vi "624WPI_DashboardGetInfo.vi"(7 "Vision":u16(ring) items=["Camera Off", "USB Camera SW", "USB Camera HW", "IP Camera"], 8 "Binding Refnum":refnum<notifier>, 9 "Window Mode Notifier":refnum<notifier>, 11 "TCP Cnx":refnum<k5>) -> (0 "Power and Errors":T2, 1 "Robot Metrics":T3, 2 "Status Info":T5, 3 "Control Info":T4 {"Team Station" items=["Red 1", "Red 2", "Red 3", "Blue 1", "Blue 2", "Blue 3"]}, 4 "Robot Mode":T1(ring), 5 "Process?":bool, 6 "Custom Dashboard Data":string)   [LabVIEW 2015]
uses:
  Dashboard Hijack Data.ctl
  <vilib>/Rock Robotics/WPI/Dashboard/WPI_DashboardLogging Global.vi
panel:
  # "CAN Metrics\nJS HID Outputs\nFree Mem"
  # "Need to merge in TCP info too"
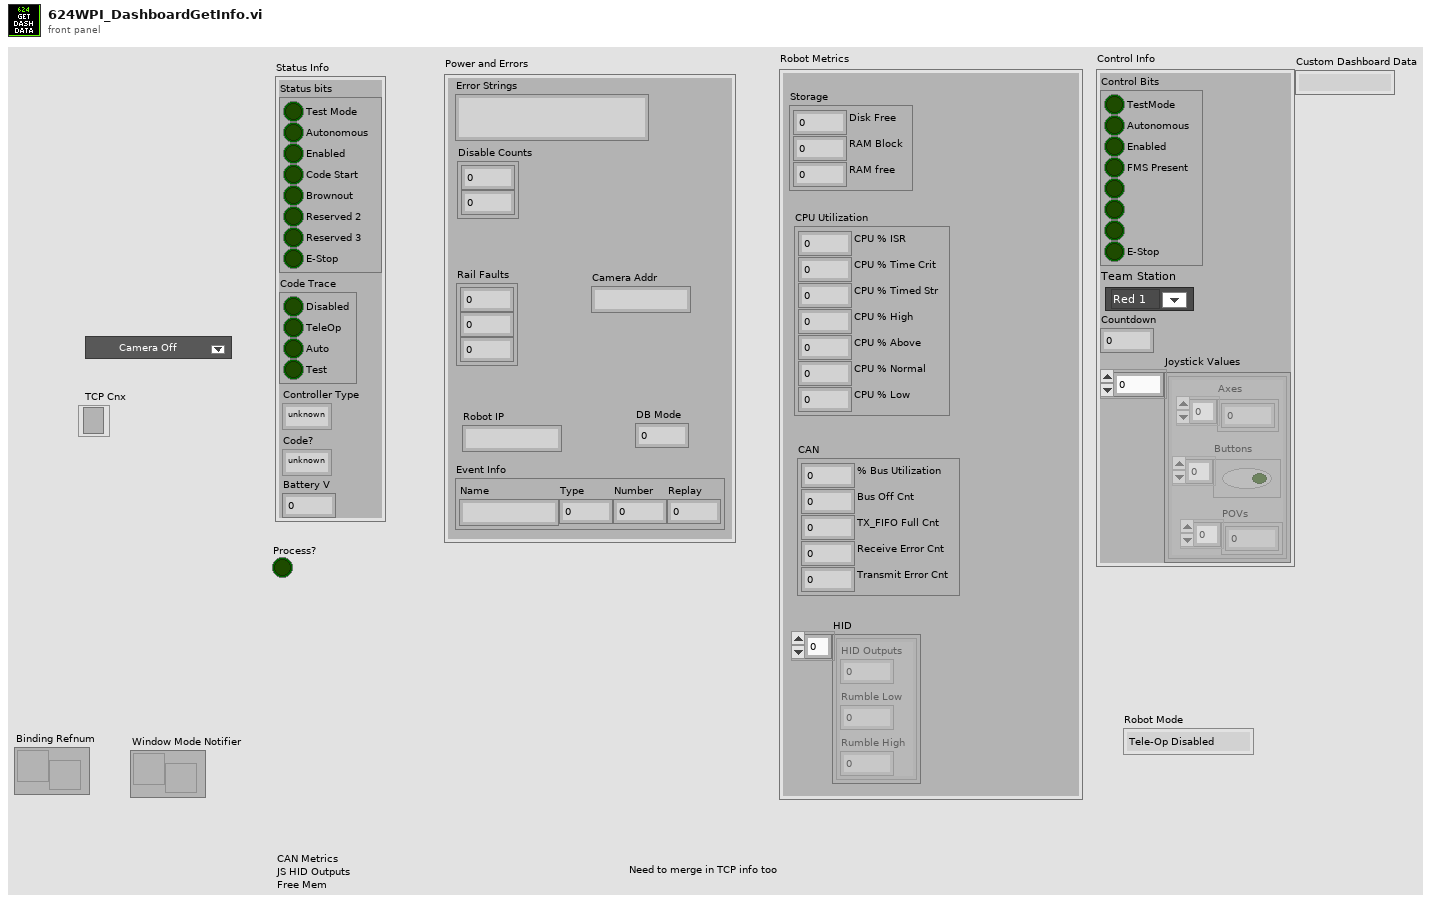
[diagram p1: front panel]
types:
  T1 = enum8{"Tele-Op Disabled", "Tele-Op Enabled", "Auto Disabled", "Auto Enabled", "Test Disabled", "Test Enabled", "Disconnected", "No Code", "E-Stop"}
  T2 = cluster{"Error Strings":string, "Disable Counts":cluster{u16, u16}, "Rail Faults":cluster{u16, u16, u16}, "Robot IP":string, "DB Mode":u8, "Event Info":cluster{"Name":string, "Type":u8, "Number":u16, "Replay":u8}, "Camera Addr":string}
  T3 = cluster{"Storage":cluster{"Disk Free":u64, "RAM Block":u32, "RAM free":u32}, "CPU Utilization":cluster{"CPU % ISR":sgl, "CPU % Time Crit":sgl, "CPU % Timed Str":sgl, "CPU % High":sgl, "CPU % Above":sgl, "CPU % Normal":sgl, "CPU % Low":sgl}, "CAN":cluster{"% Bus Utilization":sgl, "Bus Off Cnt":u32, "TX_FIFO Full Cnt":u32, "Receive Error Cnt":u8, "Transmit Error Cnt":u8}, "HID":cluster{"HID Outputs":u32, "Rumble Low":u16, "Rumble High":u16}[]}
  T4 = cluster{"Control Bits":cluster{"TestMode":bool, "Autonomous":bool, "Enabled":bool, "FMS Present":bool, bool, bool, bool, "E-Stop":bool}, "Team Station ":u8, "Countdown":sgl, "Joystick Values":cluster{"Axes":dbl[], "Buttons":bool[], "POVs":i16[]}[]}
  T5 = cluster{"Status bits":cluster{"Test Mode":bool, "Autonomous":bool, "Enabled":bool, "Code Start":bool, "Brownout":bool, "Reserved 2":bool, "Reserved 3":bool, "E-Stop":bool}, "Code Trace":cluster{"Disabled":bool, "TeleOp":bool, "Auto":bool, "Test":bool}, "Controller Type":enum16{"unknown", "cRIO", "roboRio"}, "Code?":enum16{"unknown", "noCode", "code"}, "Battery V":dbl}
  T6 = typedef "Dashboard Hijack Data.ctl" = cluster{"UDP Status string":string, "Extra data string":string}
  T7 = cluster{"TestMode":bool, "Autonomous":bool, "Enabled":bool, "FMS Present":bool, bool, bool, bool, "E-Stop":bool}
  T8 = enum16{"Standard", "Buffered", "CRLF", "Immediate"}
  T9 = cluster{"UDP Status":string, "TCP":string, "UDP Control":string}
  T10 = cluster{cluster{"Disk Free":u64, "RAM Block":u32, "RAM free":u32}, cluster{"CPU Load ISR":sgl, "CPU Load Time Critical Pr":sgl, "CPU Load Timed Str Pr":sgl, "CPU Load High Pr":sgl, "CPU Load Above Normal Pr":sgl, "CPU Load Normal Pr":sgl, "CPU Load Low Pr":sgl}, cluster{"% Bus Utilization":sgl, "Bus Off Cnt":u32, "TX_FIFO Full Cnt":u32, "Receive Error Cnt":u8, "Transmit Error Cnt":u8}, cluster{"HID Outputs":u32, "Rumble Low":u16, "Rumble High":u16}[]}
  T11 = cluster{"Status":cluster{"Test Mode":bool, "Autonomous":bool, "Enabled":bool, "Code Start":bool, "Brownout":bool, "Reserved 2":bool, "Reserved 3":bool, "E-Stop":bool}, cluster{bool, bool, bool, bool}, "ctrl":enum16{"unknown", "cRIO", "roboRio"}, "code?":enum16{"unknown", "noCode", "code"}, dbl}
  T12 = cluster{"Boolean array":cluster{"Boolean array[0]":bool, "Boolean array[1]":bool, "Boolean array[2]":bool, "Boolean array[3]":bool, "Boolean array[4]":bool, "Boolean array[5]":bool, "Boolean array[6]":bool, "Boolean array[7]":bool}, u8, "Countdown":sgl, cluster{dbl[], bool[], i16[]}[]}
  T13 = cluster{"Error Strings":string, "Disable Counts":cluster{u16, u16}, "Rail Faults":cluster{u16, u16, u16}, "Robot IP":string, "Mode":u8, "Event Info":cluster{"Name":string, "Type":u8, "Number":u16, "Replay":u8}, "Robot IP":string}
  T14 = cluster{"Boolean array[0]":bool, "Boolean array[1]":bool, "Boolean array[2]":bool, "Boolean array[3]":bool, "Boolean array[4]":bool, "Boolean array[5]":bool, "Boolean array[6]":bool, "Boolean array[7]":bool}
  T15 = typedef "Protocol Operations.ctl" = enum16{"Unknown", "Keep Alive", "Client Hello", "Version not supported", "Server Hello Complete", "Assign", "Update", "No Op", "Server Hello", "Client Hello Complete", "Update Flags", "Delete Entry", "Delete All", "RPC Exec", "RPC Response"}
  T16 = typedef "Field Data.ctl" = cluster{"Dbl":dbl, "String":string, "Type":T17, "Boolean":bool, "Sequence #":T18, "Flags":u8}
  T17 = typedef "Field Type.ctl" = enum8{"Invalid", "Bool", "Numeric", "String", "Raw", "Boolean Array", "Numeric Array", "String Array", "RPC"}
  T18 = typedef "Sequence.ctl" = u16
  T19 = cluster{"Operation":T15, "Name":string, "Field Value":T16}[]
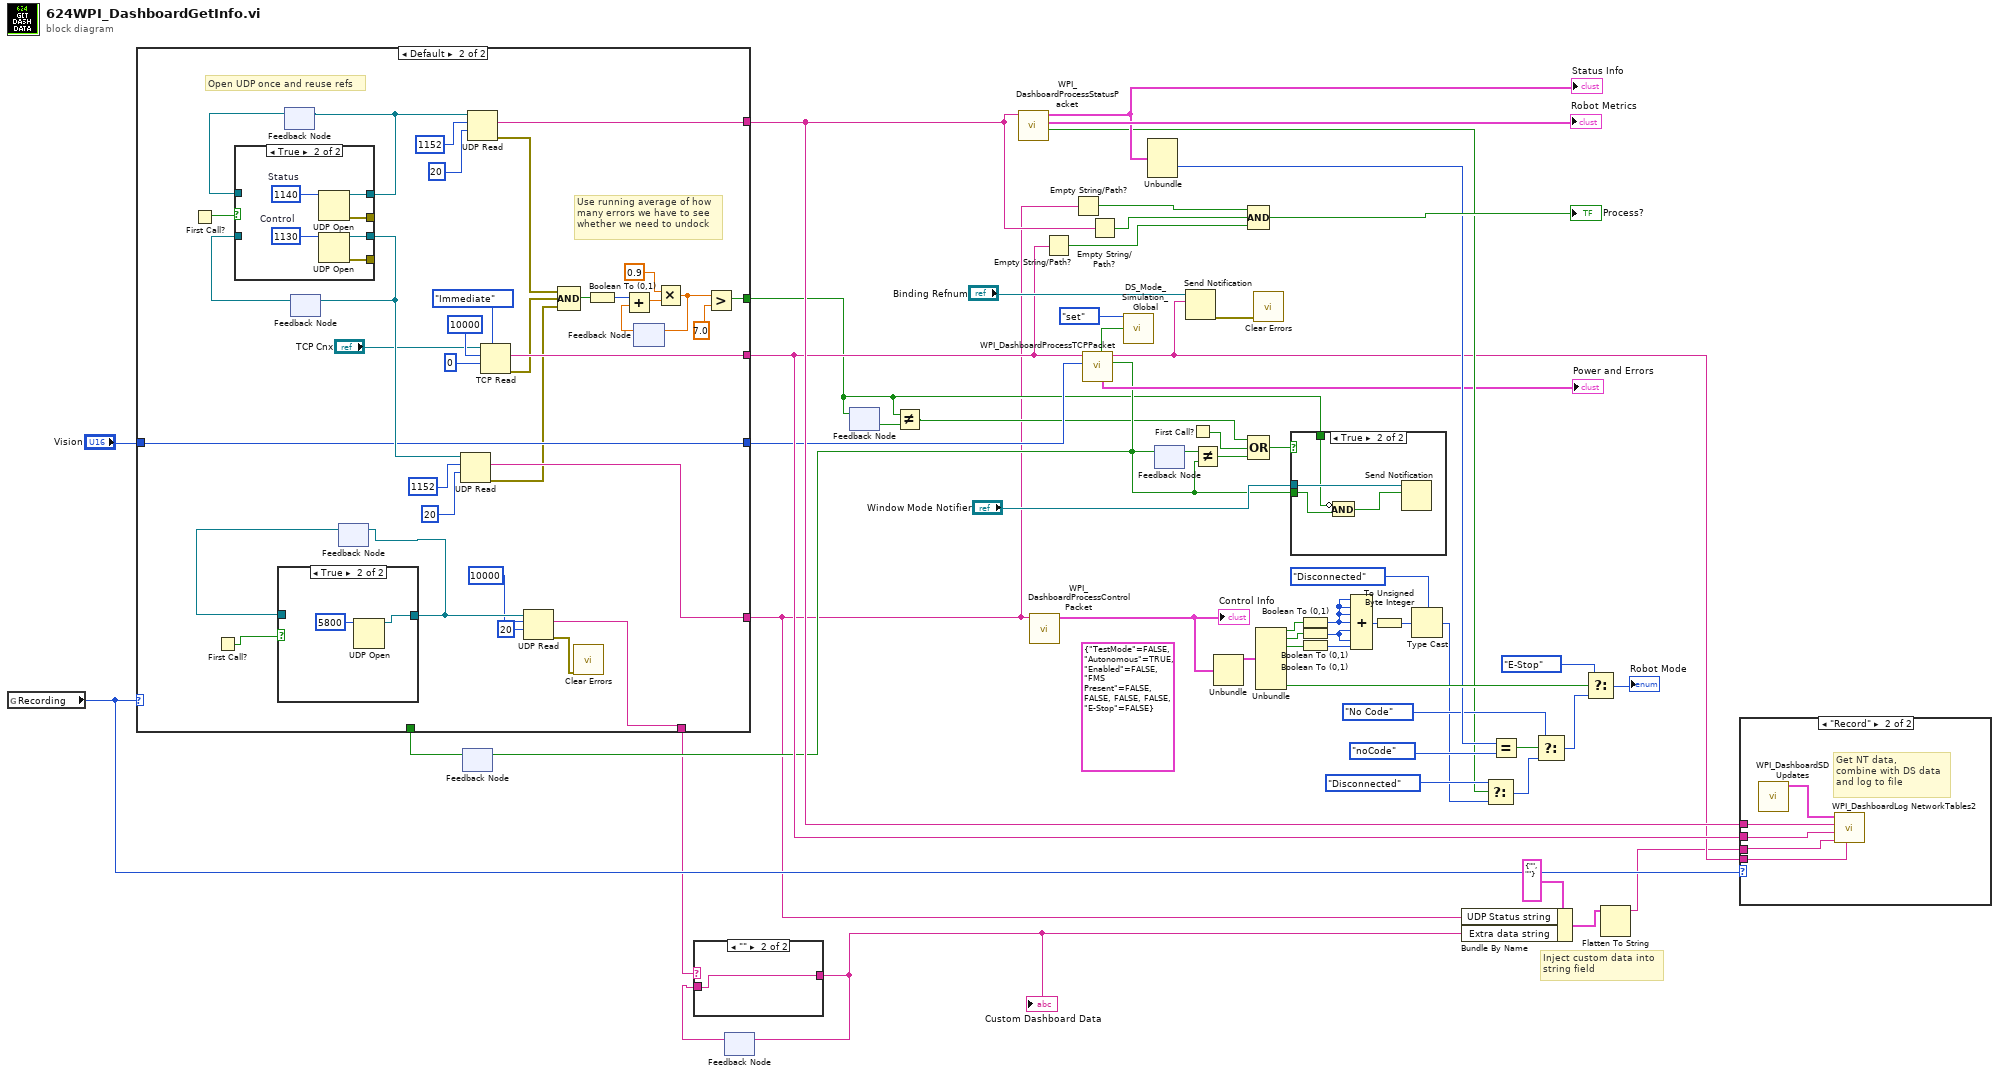
[diagram p0: block diagram]
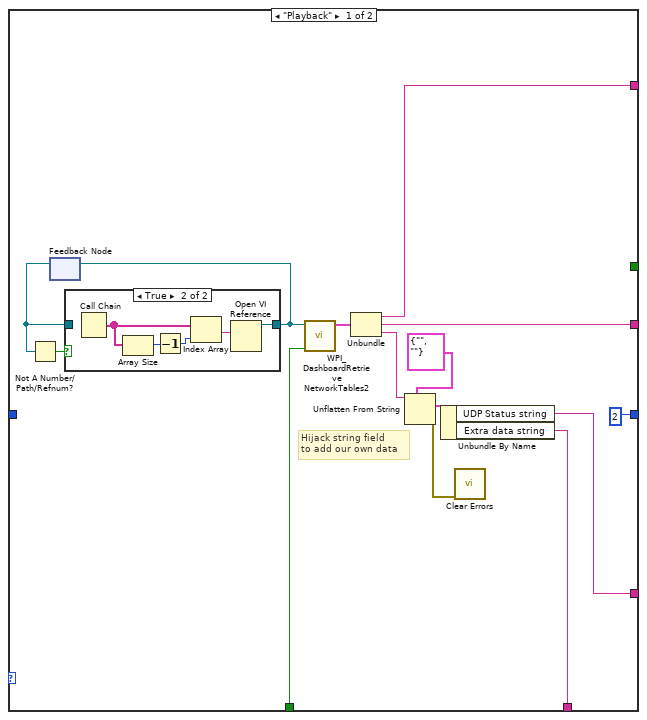
[diagram p4: hidden frame]
diagram:
  (unwired) T7 {"TestMode"=FALSE, "Autonomous"=TRUE, "Enabled"=FALSE, "FMS Present"=FALSE, FALSE, FALSE, FALSE, "E-Stop"=FALSE} ("Control Bits")
  # "Inject custom data into\nstring field"
  n1 = global read "WPI_DashboardLogging Global.vi" "Recording"() -> (w12:enum32{"Stop", "Record", "Playback"})
  n2 = feedback #1() -> (w15:bool)  [unwired: 1 in]
  n3 = case shown="Default" w12 {
    tunnel: [w60 w105] -> w7
    tunnel: [w67 w104] -> w20
    tunnel: [w66 w103] -> w19
    tunnel: w15 -> [w65 _]
    tunnel: "Vision" -> [_ w96]
    tunnel: [2 ("timeout ms (25000)") w96] -> w13
    tunnel: [_ w85] -> w11
    tunnel: [w59 w84] -> w4
    frame "Playback" {
      # "Hijack string field\nto add our own data"
      n4 = feedback #2() -> (w71:refnum<vi>)  [unwired: 1 in]
      n5 = Not A Number/Path/Refnum?(number/path/refnum=w71) -> (NaN/Path/Refnum?=w70:bool)
      n6 = case shown="True" w70 {
        tunnel: w71 -> [w72 _]
        tunnel: [w72 w76] -> w68
        frame False {
        }
        frame True {
          n7 = Call Chain() -> (call chain=w75:string[])
          n8 = Array Size(array=w75) -> (size(s)=w74:i32)
          n9 = Decrement(x=w74) -> (x-1=w73:i32)
          n10 = Index Array(array=w75, index=w73) -> (element=w77:string)
          n11 = Open VI Reference(vi path=w77) -> (vi reference=w76:refnum<vi>)  [unwired: 5 in, 1 out]
        }
      }
      n12 = feedback-in #2(w68) -> ()
      n13 = call <vilib>:"WPI_DashboardRetrieve NetworkTables2.vi"("Docked Window"=w65, "VI Refnum"=w68) -> ("Strings"=w69:T9)  [unwired: 9 in]
      n14 = Unbundle(w69) -> ("UDP Status"=w67:string, "TCP"=w66:string, "UDP Control"=w63:string)
      n15 = Unflatten From String(type=T6 {"UDP Status string"="", "Extra data string"=""} ("Dashboard Data Hijack"), binary string=w63) -> (value=w61:T6, error out=w58:errorcluster)  [unwired: 3 in, 1 out]
      n16 = Unbundle By Name(w61) -> ("UDP Status string"=w60:string, "Extra data string"=w59:string)
      n17 = call <vilib>:"Clear Errors.vi"("error in (no error)"=w58) -> ()  [unwired: 5 in, 2 out]
    }
    frame Default {
      # "Use running average of how\nmany errors we have to see\nwhether we need to undock"
      # "Open UDP once and reuse refs"
      n18 = First Call?() -> (First Call?: T/F=w102:bool)
      n19 = First Call?() -> (First Call?: T/F=w81:bool)
      n20 = feedback #3() -> (w100:refnum<k16>)  [unwired: 1 in]
      n21 = feedback #4() -> (w98:refnum<k16>)  [unwired: 1 in]
      n22 = case shown="True" w102 {
        tunnel: [w117 w121] -> w101
        tunnel: [_ w120] -> _
        tunnel: [w116 w119] -> w99
        tunnel: [_ w118] -> _
        tunnel: w100 -> [w117 _]
        tunnel: w98 -> [w116 _]
        frame False {
        }
        frame True {
          w122 = u16 1130  # Control
          w123 = u16 1140  # Status
          n23 = UDP Open(11:w123) -> (port=w121:refnum<k16>, 0:w120:errorcluster)  [unwired: 2 in, 3 out]
          n24 = UDP Open(11:w122) -> (port=w119:refnum<k16>, 0:w118:errorcluster)  [unwired: 2 in, 3 out]
        }
      }
      n25 = feedback-in #3(w101) -> ()
      n26 = feedback-in #4(w99) -> ()
      n27 = feedback #5() -> (w83:refnum<k16>)  [unwired: 1 in]
      n28 = case shown="True" w81 {
        tunnel: [w113 w114] -> w82
        tunnel: w83 -> [w113 _]
        frame False {
        }
        frame True {
          n29 = UDP Open(11:u16 5800 ("port")) -> (port=w114:refnum<k16>)  [unwired: 4 in, 2 out]
        }
      }
      n30 = feedback-in #5(w82) -> ()
      n31 = UDP Read(connection ID=w99, max size (548)=1152, timeout ms (25000)=20 ("length (rest)")) -> (data out=w105:string, error out=w93:errorcluster)  [unwired: 1 in, 3 out]
      n32 = UDP Read(connection ID=w101, max size (548)=1152, timeout ms (25000)=20 ("length (rest)")) -> (data out=w104:string, error out=w95:errorcluster)  [unwired: 1 in, 3 out]
      n33 = TCP Read(connection ID="TCP Cnx", bytes to read=10000 ("timeout ms (25000)"), 7:T8."Immediate" ("mode (standard)"), 9:0 ("timeout ms (25000)")) -> (data out=w103:string, error out=w94:errorcluster)  [unwired: 1 in, 1 out]
      n34 = UDP Read(connection ID=w82, max size (548)=10000, timeout ms (25000)=20) -> (data out=w84:string, error out=w79:errorcluster)  [unwired: 1 in, 3 out]
      n35 = Compound Arithmetic op=AND(w95, w94, w93) -> (w92:bool)
      n36 = call <vilib>:"Clear Errors.vi"("error in (no error)"=w79) -> ()  [unwired: 5 in, 2 out]
      n37 = Boolean To (0,1)(Boolean=w92) -> (0, 1=w91:i16)
      n38 = feedback #6() -> (w90:dbl)  [unwired: 1 in]
      n39 = Add(x=w91, y=w90) -> (x+y=w89:dbl)
      n40 = Multiply(x=0.9 ("timeout ms (25000)"), y=w89) -> (x*y=w87:dbl)
      n41 = feedback-in #6(w87) -> ()
      n42 = Greater?(x=w87, y=7.0 ("timeout ms (25000)")) -> (0:w85:bool)
    }
  }
  n43 = feedback #7() -> (w3:string)  [unwired: 1 in]
  n44 = case shown="\"\"" w4 {
    selector: w4 -> [w124 _]
    tunnel: [w124 w125] -> w2
    tunnel: w3 -> [_ w125]
    frame Default {
    }
    frame "" {
    }
  }
  "Custom Dashboard Data" <- w2
  n45 = feedback-in #7(w2) -> ()
  n46 = feedback #8() -> (w10:bool)  [unwired: 1 in]
  n47 = feedback-in #8(w11) -> ()
  n48 = Not Equal?(x=w11, y=w10) -> (x != y?=w9:bool)
  n49 = call <vilib>:"WPI_DashboardProcessStatusPacket.vi"("data in"=w20) -> ("Disconnected"=w23:bool, "Robot Metrics"=→"Robot Metrics":T10, "Status Cluster"=w37:T11)  [unwired: 8 in]
  "Status Info" <- w37
  n50 = call <vilib>:"WPI_DashboardProcessControlPacket.vi"("data in"=w7) -> ("Control Info"=w45:T12)  [unwired: 10 in]
  "Control Info" <- w45
  n51 = Empty String/Path?(string/path=w19) -> (empty?=w55:bool)
  n52 = Empty String/Path?(string/path=w7) -> (empty?=w53:bool)
  n53 = call <vilib>:"WPI_DashboardProcessTCPPacket.vi"("Vision"=w13, "data in"=w19) -> ("Docked"=w16:bool, "Robot IP"=w17:string, "Power and Errors"=→"Power and Errors":T13, "Simulated"=w21:bool)  [unwired: 5 in, 1 out]
  n54 = feedback-in #1(w16) -> ()
  n55 = Empty String/Path?(string/path=w20) -> (empty?=w54:bool)
  n56 = call <vilib>:"DS_Mode_Simulation_Global.vi"("menu"=enum16{"set", "get"}."set", "simulated? in"=w21) -> ()  [unwired: 12 in, 2 out]
  n57 = Unbundle(w37) -> ("code?"=w33:enum16{"unknown", "noCode", "code"})  [unwired: 4 out]
  n58 = feedback #9() -> (w48:bool)  [unwired: 1 in]
  n59 = feedback-in #9(w16) -> ()
  n60 = Send Notification(notification=w17, notifier="Binding Refnum") -> (error out=w1:errorcluster)  [unwired: 1 in, 1 out]
  n61 = First Call?() -> (First Call?: T/F=w50:bool)
  n62 = Not Equal?(x=w48, y=w16) -> (x != y?=w49:bool)
  n63 = Unbundle(w45) -> ("Boolean array"=w44:T14)  [unwired: 3 out]
  n64 = Compound Arithmetic op=AND(w53, w54, w55) -> (→"Process?":bool)
  n65 = Compound Arithmetic op=OR(w9, w50, w49) -> (w51:bool)
  n66 = call <vilib>:"Clear Errors.vi"("error in (no error)"=w1) -> ()  [unwired: 5 in, 2 out]
  n67 = Unbundle(w44) -> ("Boolean array[0]"=w39:bool, "Boolean array[1]"=w40:bool, "Boolean array[2]"=w42:bool, "Boolean array[7]"=w36:bool)  [unwired: 4 out]
  n68 = case shown="True" w51 {
    tunnel: "Window Mode Notifier" -> [_ w129]
    tunnel: w16 -> [_ w127]
    tunnel: w11 -> [_ w128]
    frame False {
    }
    frame True {
      n69 = Compound Arithmetic op=AND(invert w128, w127) -> (w126:bool)
      n70 = Send Notification(notification=w126, notifier=w129) -> ()  [unwired: 1 in, 2 out]
    }
  }
  n71 = Boolean To (0,1)(Boolean=w39) -> (0, 1=w38:i16)
  n72 = Boolean To (0,1)(Boolean=w40) -> (0, 1=w41:i16)
  n73 = Boolean To (0,1)(Boolean=w42) -> (0, 1=w43:i16)
  n74 = Compound Arithmetic op=ADD(w38, w38, w38, w38, w41, w41, w43) -> (w27:i16)
  n75 = To Unsigned Byte Integer(number=w27) -> (unsigned 8bit integer=w22:u8)
  n76 = Type Cast(type=T1."Disconnected" ("Mode"), x=w22) -> (*(type *) &x=w26:T1)
  n77 = Bundle By Name(cluster=T6 {"UDP Status string"="", "Extra data string"=""} ("Dashboard Data Hijack"), "UDP Status string"=w7, "Extra data string"=w2) -> (w6:T6)
  n78 = Select(t=T1."Disconnected" ("Mode"), s=w23, f=w26) -> (s? t:f=w29:T1)
  n79 = Equal?(x=w33, y=enum16{"unknown", "noCode", "code"}."noCode" ("code?")) -> (x = y?=w32:bool)
  n80 = Select(t=T1."No Code" ("Mode"), s=w32, f=w29) -> (s? t:f=w31:T1)
  n81 = Select(t=T1."E-Stop" ("Mode"), s=w36, f=w31) -> (s? t:f=→"Robot Mode":T1)
  n82 = Flatten To String(anything=w6) -> (data string=w5:string)  [unwired: 3 in, 2 out]
  n83 = case shown="\"Record\"" w12 {
    tunnel: w20 -> [_ w131]
    tunnel: w19 -> [_ w132]
    tunnel: w5 -> [_ w133]
    tunnel: w17 -> [_ w130]
    frame Default {
    }
    frame "Record" {
      # "Get NT data,\ncombine with DS data\nand log to file"
      n84 = call <vilib>:"WPI_DashboardSD Updates.vi"() -> ("Collected Data"=w134:T19)  [unwired: 11 in]
      n85 = call <vilib>:"WPI_DashboardLog NetworkTables2.vi"("Robot IP"=w130, "UDP Control"=w133, "TCP"=w132, "UDP Status"=w131, "NT Data Values"=w134) -> ()  [unwired: 7 in]
    }
  }
